vi "ProbeObjectKernel.vi"(0 "ObjectStatus":refnum<vi>, 1 "Ref":variant, 2 "ObjAttribute":string, 3 "ClassAttribute":string, 4 "ClassProvider":T1, 5 "error in":errorcluster, 6 "Mode(Get)":enum16{"Get", "Set", "Delete"}(ring)) -> (15 "DebuggerOut":T2, 19 "error out":errorcluster)   [LabVIEW 2020, in "ClassWriterGOOP300.lvclass"]
uses:
  <resource>/Framework/Providers/Open_GDS/ClassProviders/Provider_EndevoGOOP300/ClassWriterGOOP300_class/ClassWriterGOOP300.lvclass
  <resource>/Framework/Providers/Open_GDS/ClassProviders/Common/LvClass_class/GDSLvClass_ProviderTypes.ctl
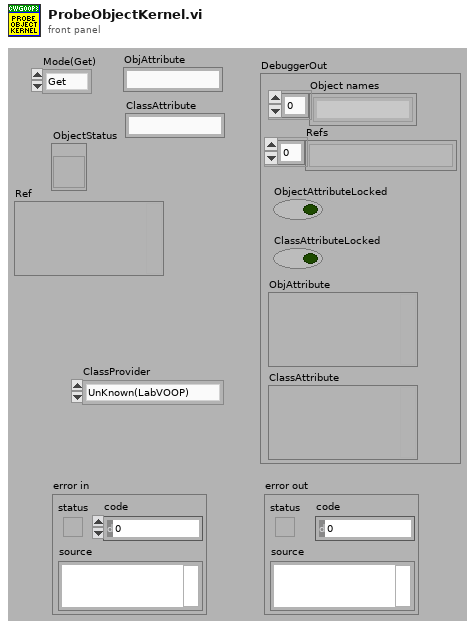
[diagram p1: front panel]
types:
  T1 = typedef "GDSLvClass_ProviderTypes.ctl" = enum16{"UnKnown(LabVOOP)", "Native", "EndevoGOOP3", "OpenG(RootObject)", "OpenG(OpenG_Object)", "EndevoGOOP4", "JKI1"}
  T2 = cluster{"Object names":string[], "Refs":variant[], "ObjectAttributeLocked":bool, "ClassAttributeLocked":bool, "ObjAttribute":variant, "ClassAttribute":variant}
  T3 = cluster{"Mode":enum16{"Get", "Set", "Delete"}, "Ref":variant, "ObjAttribute":string, "ClassAttribute":string}
  T4 = cluster{"Object names":string[], "Refs":i32[], "ObjectAttributeLocked":bool, "ClassAttributeLocked":bool, "ObjAttribute":variant, "ClassAttribute":variant}
  T5 = cluster{"Object names":string[], "Refs":variant, "ObjectAttributeLocked":bool, "ClassAttributeLocked":bool, "ObjAttribute":variant, "ClassAttribute":variant}
  T6 = cluster{"Mode":enum16{"Get", "Set", "Delete"}, "Ref":i32, "ObjAttribute":string, "ClassAttribute":string}
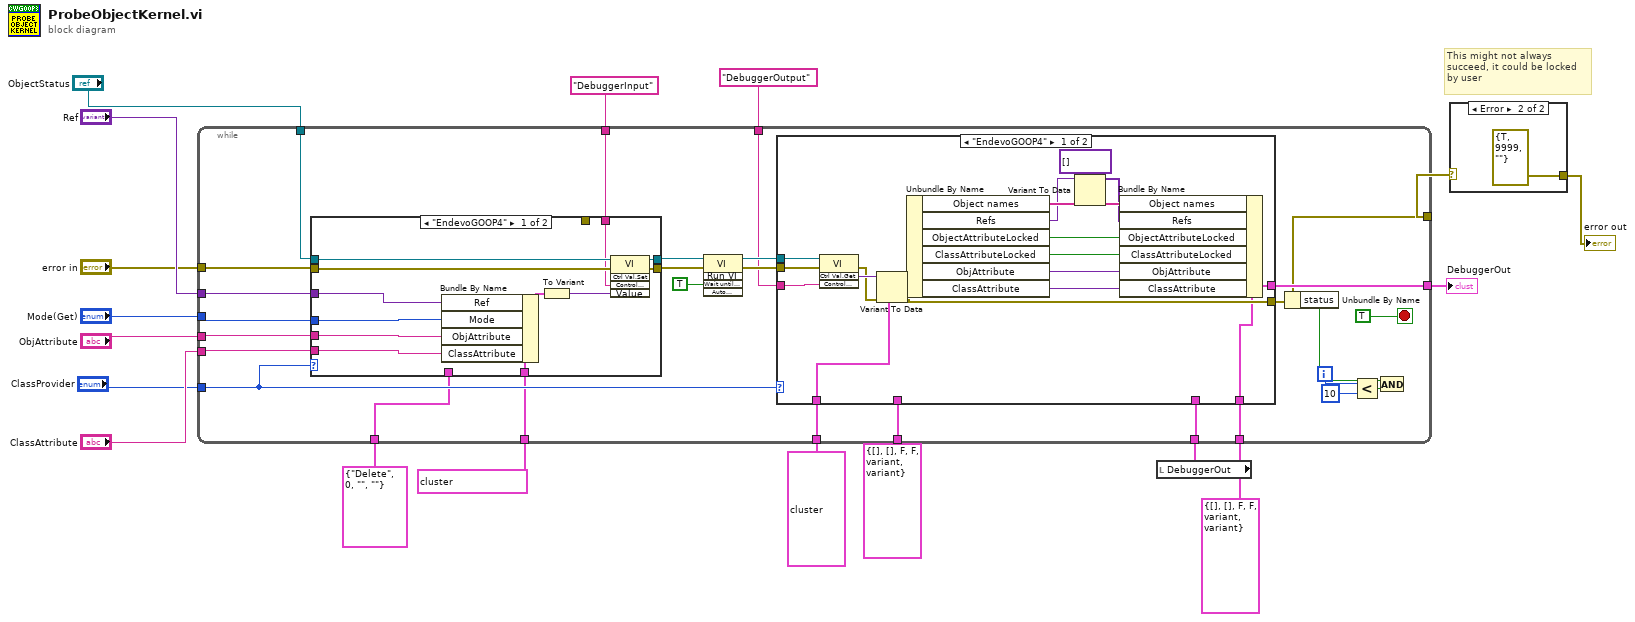
[diagram p0: block diagram]
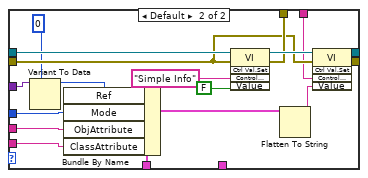
[diagram p3: hidden frame]
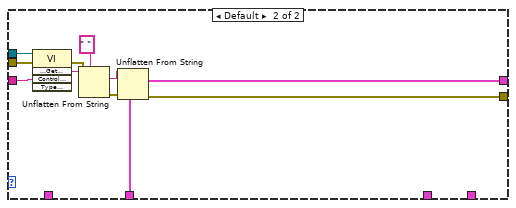
[diagram p4: hidden frame]
diagram:
  # "This might not always\nsucceed, it could be locked\nby user"
  n1 = local read "DebuggerOut"() -> (w14:T2)
  n2 = while {
    tunnel: "ObjectStatus" -> [w32]
    tunnel: [w39] -> w18
    tunnel: w14 -> [w36]
    tunnel: T6 {"Mode"=enum."Delete", "Ref"=0, "ObjAttribute"="", "ClassAttribute"=""} ("DebuggerIn") -> [w25]
    tunnel: "error in" -> [w31]
    tunnel: [w35] -> w9
    tunnel: "Ref" -> [w21]
    tunnel: "Mode(Get)" -> [w24]
    tunnel: "ObjAttribute" -> [w23]
    tunnel: "ClassAttribute" -> [w22]
    tunnel: "ClassProvider" -> [w26]
    tunnel: T4 {"Object names"=[], "Refs"=[], "ObjectAttributeLocked"=FALSE, "ClassAttributeLocked"=FALSE, "ObjAttribute"=variant, "ClassAttribute"=variant} ("DebuggerOut") -> [w30]
    tunnel: T5 {"Object names"=[], "Refs"=variant, "ObjectAttributeLocked"=FALSE, "ClassAttributeLocked"=FALSE, "ObjAttribute"=variant, "ClassAttribute"=variant} ("DebuggerOut") -> [w29]
    tunnel: "DebuggerInput" ("Control Name") -> [w28]
    tunnel: "DebuggerOutput" ("Control Name") -> [w27]
    tunnel: T3 {"Mode"=enum."Delete", "Ref"=variant, "ObjAttribute"="", "ClassAttribute"=""} ("DebuggerIn") -> [w20]
    tunnel: T2 {"Object names"=[], "Refs"=[], "ObjectAttributeLocked"=FALSE, "ClassAttributeLocked"=FALSE, "ObjAttribute"=variant, "ClassAttribute"=variant} ("DebuggerOut") -> [w19]
    i -> [w34]
    stop <- TRUE stop-if-true
    n3 = case shown="\"EndevoGOOP4\"" w26 {
      tunnel: [w53 w75] -> w38
      tunnel: [w54 w74] -> w37
      tunnel: w32 -> [w57 w70]
      tunnel: [_ w68] -> _
      tunnel: w31 -> [w56 w67]
      tunnel: w28 -> [w55 w66]
      tunnel: w25 -> [_ w64]
      tunnel: w24 -> [w51 w63]
      tunnel: w23 -> [w50 w62]
      tunnel: w22 -> [w49 w61]
      tunnel: w21 -> [w48 w58]
      tunnel: w20 -> [w52 _]
      frame "EndevoGOOP4" {
        n4 = Bundle By Name(cluster=w52, "Ref"=w48, "Mode"=w51, "ObjAttribute"=w50, "ClassAttribute"=w49) -> (w47:T3)
        n5 = To Variant(anything=w47) -> (Variant=w46:variant)
        n6 = invoke class="VI" method="Ctrl Val.Set"(reference=w57, error in=w56, "Control Name"=w55, "Value"=w46) -> (reference out=w54:refnum<vi>, error out=w53:errorcluster)  [unwired: 1 in, 3 out]
      }
      frame Default {
        n7 = Variant To Data(type=0 ("Ref"), Variant=w58) -> (data=w59:i32)  [unwired: 1 in, 1 out]
        n8 = Bundle By Name(cluster=w64, "Ref"=w59, "Mode"=w63, "ObjAttribute"=w62, "ClassAttribute"=w61) -> (w65:T6)
        n9 = invoke class="VI" method="Ctrl Val.Set"(reference=w70, error in=w67, "Control Name"="Simple Info", "Value"=FALSE) -> (reference out=w69:refnum<vi>, error out=w68:errorcluster)  [unwired: 1 in, 3 out]
        n10 = Flatten To String(anything=w65) -> (data string=w73:string)  [unwired: 3 in, 2 out]
        n11 = invoke class="VI" method="Ctrl Val.Set"(reference=w69, error in=w67, "Control Name"=w66, "Value"=w73) -> (reference out=w74:refnum<vi>, error out=w75:errorcluster)  [unwired: 1 in, 3 out]
      }
    }
    n12 = invoke class="VI" method="Run VI"(reference=w37, error in=w38, "Wait until done"=TRUE ("Wait Until Done")) -> (reference out=w44:refnum<vi>, error out=w43:errorcluster)  [unwired: 2 in, 3 out]
    n13 = case shown="\"EndevoGOOP4\"" w26 {
      tunnel: w44 -> [w93 w104]
      tunnel: w43 -> [w92 w103]
      tunnel: w27 -> [w91 w102]
      tunnel: [w76 w101] -> w39
      tunnel: w36 -> [_ _]
      tunnel: [w87 w95] -> w35
      tunnel: w30 -> [_ w94]
      tunnel: w29 -> [w89 _]
      tunnel: w19 -> [w85 _]
      frame "EndevoGOOP4" {
        n14 = invoke class="VI" method="Ctrl Val.Get"(reference=w93, error in=w92, "Control Name"=w91) -> (error out=w88:errorcluster, "Get Control Value Variant"=w90:variant)  [unwired: 1 in, 2 out]
        n15 = Variant To Data(error in=w88, type=w89, Variant=w90) -> (data=w86:T5, error out=w87:errorcluster)
        n16 = Unbundle By Name(w86) -> ("Object names"=w84:string[], "Refs"=w83:variant, "ObjectAttributeLocked"=w80:bool, "ClassAttributeLocked"=w79:bool, "ObjAttribute"=w78:variant, "ClassAttribute"=w77:variant)
        n17 = Variant To Data(type=variant[] [] ("Refs"), Variant=w83) -> (data=w81:variant[])  [unwired: 1 in, 1 out]
        n18 = Bundle By Name(cluster=w85, "Object names"=w84, "Refs"=w81, "ObjectAttributeLocked"=w80, "ClassAttributeLocked"=w79, "ObjAttribute"=w78, "ClassAttribute"=w77) -> (w76:T2)
      }
      frame Default {
        n19 = invoke class="VI" method="Ctrl Val.Get (Deprecated)"(reference=w104, error in=w103, "Control Name"=w102) -> (error out=w97:errorcluster, "Get Control Value"=w100:string)  [unwired: 2 in, 3 out]
        n20 = Unflatten From String(type=" ", binary string=w100, error in (no error)=w97) -> (value=w98:string, error out=w96:errorcluster)  [unwired: 2 in, 1 out]
        n21 = Unflatten From String(type=w94, binary string=w98, error in (no error)=w96) -> (value=w101:T4, error out=w95:errorcluster)  [unwired: 2 in, 1 out]
      }
    }
    n22 = Unbundle By Name(w35) -> ("status"=w41:bool)
    n23 = Less?(x=w34, y=10) -> (x < y?=w40:bool)
    n24 = And(x=w41, y=w40) -> ()  [unwired: 1 out]
  }
  "DebuggerOut" <- w18
  n25 = case shown="Error" w9 {
    selector: w9 -> [w105 _]
    tunnel: [w105 errorcluster {"status"=TRUE, "code"=9999, "source"=""} ("error out")] -> w8
    frame No Error {
    }
    frame Error {
    }
  }
  "error out" <- w8
